vi "GetThisMachine.vi"() -> (3 "ThisMachine":string)   [LabVIEW 2021, in "ProligentXMLGenerator.lvlib"]
uses:
  ProligentXMLGenerator.lvlib
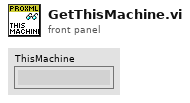
[diagram p1: front panel]
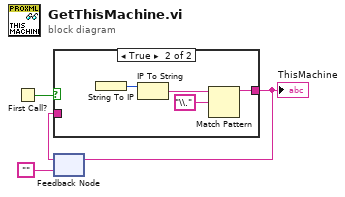
[diagram p0: block diagram]
diagram:
  n1 = First Call?() -> (First Call?: T/F=w4:bool)
  n2 = feedback #1("") -> (w2:string)
  n3 = case shown="True" w4 {
    tunnel: [w5 w9] -> w3
    tunnel: w2 -> [w5 _]
    frame False {
    }
    frame True {
      n4 = String To IP() -> (0:w8:u32)  [unwired: 1 in]
      n5 = IP To String(2:w8) -> (0:w6:string)  [unwired: 1 in]
      n6 = Match Pattern(string=w6, regular expression="\\.") -> (before substring=w9:string)  [unwired: 1 in, 3 out]
    }
  }
  "ThisMachine" <- w3
  n7 = feedback-in #1(w3) -> ()
